vi "largeurmi-haut.vi"(2 "Y":dbl[](array[numeric]), 3 "X":dbl[](array[numeric])) -> (1 "FWHM":dbl)   [LabVIEW 2014]
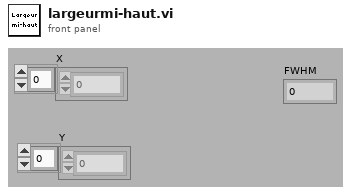
[diagram p1: front panel]
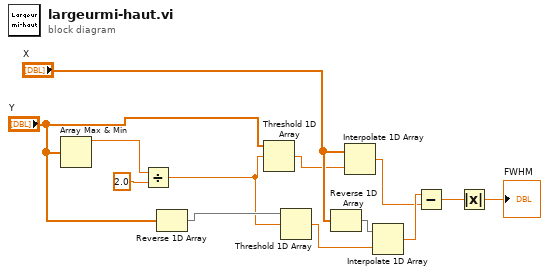
[diagram p0: block diagram]
diagram:
  n1 = Array Max & Min(array="Y") -> (max value=w3:dbl)  [unwired: 3 out]
  n2 = Divide(x=w3, y=2.0) -> (x/y=w10:dbl)
  n3 = Reverse 1D Array(array="Y") -> (reversed array=w11:dbl[])
  n4 = Threshold 1D Array(2:w10, 3:"Y") -> (0:w7:dbl)  [unwired: 1 in]
  n5 = Threshold 1D Array(2:w10, 3:w11) -> (0:w6:dbl)  [unwired: 1 in]
  n6 = Reverse 1D Array(array="X") -> (reversed array=w8:dbl[])
  n7 = Interpolate 1D Array(1:w7, 2:"X") -> (0:w4:dbl)
  n8 = Interpolate 1D Array(1:w6, 2:w8) -> (0:w5:dbl)
  n9 = Subtract(x=w5, y=w4) -> (x-y=w2:dbl)
  n10 = Absolute Value(x=w2) -> (abs(x)=→"FWHM":dbl)
